vi "get_library_icon.vi"(8 "error in (no error)":errorcluster, 11 "Icon XML line":string) -> (0 "error out":errorcluster, 3 "Icon":picture)   [LabVIEW 2020]
doc: "Created by Ryan Pacini"
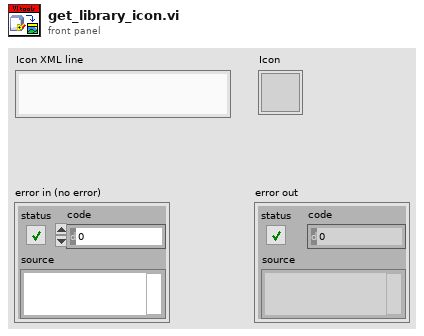
[diagram p1: front panel]
types:
  T1 = cluster{"image type":i32, "image depth":i32, "image":u8[], "mask":u8[], "colors":u32[], "Rectangle":cluster{"left":i16, "top":i16, "right":i16, "bottom":i16}}
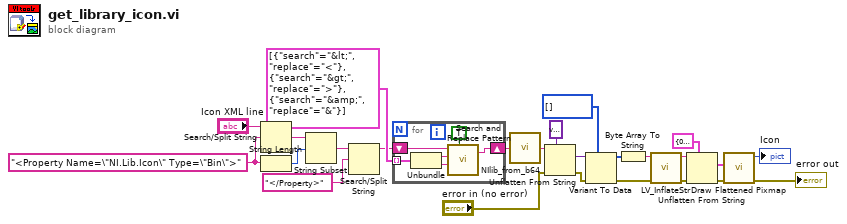
[diagram p0: block diagram]
diagram:
  w21 = "<Property Name=\"NI.Lib.Icon\" Type=\"Bin\">" ("search string/char (-)")
  n1 = Search/Split String(string="Icon XML line", search string/char (-)=w21) -> (match + rest of string=w24:string)  [unwired: 1 in, 2 out]
  n2 = String Length(string=w21) -> (length=w23:i32)
  n3 = String Subset(string=w24, offset (0)=w23) -> (substring=w22:string)  [unwired: 1 in]
  n4 = Search/Split String(string=w22, search string/char (-)="</Property>") -> (substring before match=w7:string)  [unwired: 1 in, 2 out]
  n5 = for {
    shift-right: [w25] -> w6
    shift-left: w7 -> [w30]
    tunnel: cluster{"search":string, "replace":string}[] [{"search"="&lt;", "replace"="<"}, {"search"="&gt;", "replace"=">"}, {"search"="&amp;", "replace"="&"}] -> [w28] mode=indexing
    n6 = Unbundle(w28) -> ("search"=w27:string, "replace"=w26:string)
    n7 = call <vilib>:"Search and Replace Pattern.vi"("string"=w30, "regular expression (\"\")"=w27, "replace string (\"\")"=w26, "replace all? (F)"=TRUE) -> ("result string"=w25:string)  [unwired: 1 in, 1 out]
  }
  n8 = call "NIlib_from_b64.vi"("base64 in"=w6) -> ("string out"=w5:string)
  n9 = Unflatten From String(type=variant ("variant"), binary string=w5, error in (no error)="error in (no error)") -> (value=w15:variant, error out=w16:errorcluster)  [unwired: 2 in, 1 out]
  n10 = Variant To Data(error in=w16, type=u8[] [], Variant=w15) -> (data=w13:u8[], error out=w3:errorcluster)
  n11 = Byte Array To String(unsigned byte array=w13) -> (string=w4:string)
  n12 = call "LV_InflateStr.vi"("error in (no error)"=w3, "Deflated string with size header"=w4) -> ("error out"=w2:errorcluster, "Inflated string"=w1:string)  [unwired: 8 in]
  n13 = Unflatten From String(type=T1 {"image type"=0, "image depth"=0, "image"=[], "mask"=[], "colors"=[], "Rectangle"={"left"=0, "top"=0, "right"=0, "bottom"=0}} ("image data"), binary string=w1, error in (no error)=w2) -> (value=w11:T1, error out=→"error out":errorcluster)  [unwired: 2 in, 1 out]
  n14 = call <vilib>:"Draw Flattened Pixmap.vi"("image data"=w11) -> ("new picture"=→"Icon":picture)  [unwired: 8 in]
